vi "Build Home HTML.vi"(7 "Volatus:VolatusAPI":refnum<class "VolatusAPI.lvclass">, 8 "error in (no error)":errorcluster, 11 "HomeHTTPController in":refnum<class "HomeHTTPController.lvclass">) -> (0 "error out":errorcluster, 2 "Home HTML":string, 3 "HomeHTTPController out":refnum<class "HomeHTTPController.lvclass">)   [LabVIEW 2020, in "Volatus.lvlib" / "HomeHTTPController.lvclass"]
uses:
  HomeHTTPController.lvclass
  VolatusAPI/VolatusAPI.lvclass
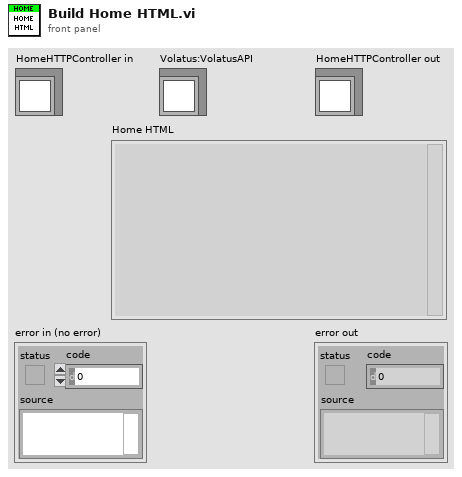
[diagram p1: front panel]
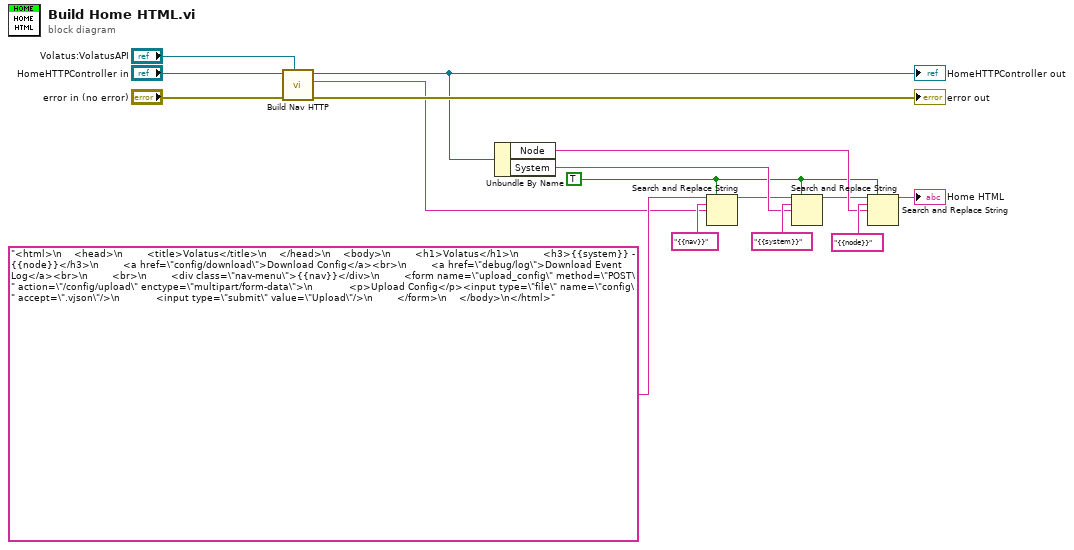
[diagram p0: block diagram]
diagram:
  w5 = TRUE ("replace all? (F)")
  n1 = call "Build Nav HTTP.vi"("VolatusAPI"="Volatus:VolatusAPI", "error in (no error)"="error in (no error)", "HomeHTTPController in"="HomeHTTPController in") -> ("error out"=→"error out":errorcluster, "Nav HTTP"=w2:string, "HomeHTTPController out"=w4:refnum<class "HomeHTTPController.lvclass">)  [unwired: 6 in]
  "HomeHTTPController out" <- w4
  n2 = Unbundle By Name(w4) -> ("Node"=w11:string, "System"=w13:string)
  n3 = Search and Replace String(replace all?=w5, input string="<html>\n    <head>\n        <title>Volatus</title>\n    </head>\n    <body>\n        <h1>Volatus</h1>\n        <h3>{{system}} - {{node}}</h3>\n        <a href=\"config/download\">Download Config</a><br>\n        <a href=\"debug/log\">Download Event Log</a><br>\n        <br>\n        <div class=\"nav-menu\">{{nav}}</div>\n        <form name=\"upload_config\" method=\"POST\" action=\"/config/upload\" enctype=\"multipart/form-data\">\n            <p>Upload Config</p><input type=\"file\" name=\"config\" accept=\".vjson\"/>\n            <input type=\"submit\" value=\"Upload\"/>\n        </form>\n    </body>\n</html>", search string="{{nav}}", replace string=w2) -> (result string=w7:string)  [unwired: 4 in, 3 out]
  n4 = Search and Replace String(replace all?=w5, input string=w7, search string="{{system}}", replace string=w13) -> (result string=w10:string)  [unwired: 4 in, 3 out]
  n5 = Search and Replace String(replace all?=w5, input string=w10, search string="{{node}}", replace string=w11) -> (result string=→"Home HTML":string)  [unwired: 4 in, 3 out]
